vi "Init Galvo Commmand.vi"(8 "error in (no error)":errorcluster) -> (0 "error out":errorcluster)   [LabVIEW 2018]
uses:
  Controls/FGV Actions.ctl
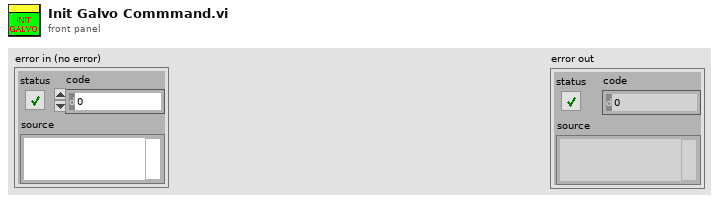
[diagram p1: front panel]
types:
  T1 = enum16{"Configure channels", "Write Scan Pattern", "Start Galvo Task", "Is Task Done?", "Stop Galvo", "Uninit", "Init: Calc scan pattern"}
  T2 = typedef "FGV Actions.ctl" = enum16{"Init", "Set", "Get", "Clear"}
  T3 = typedef "System Parameters.ctl" = cluster{"Optical Parameters":T4, "Vibratome":T5, "Table Stages":T6, "Imaging Parameter":T9, "Galvo HW Parameters":cluster{"Analog Out Channel":tag, "Min Voltage":dbl, "Max Voltage":dbl, "Pixel Clock Source":tag, "Sample Rate":dbl, "Line Clock Out Ch":tag}, "Alazar parameters":T11, "Mosaic Paramter":cluster{"X Axis":cluster{"Start [mm]":dbl, "Steps [pts]":u16, "End [mm]":dbl}, "Y Axis":cluster{"Start [mm]":dbl, "Steps [pts]":u16, "End [mm]":dbl}, "Scan Pattern":enum16{"Uni-directional", "Bi-Directional", "Spiral Out", "Spiral In"}, "Overlap Options":cluster{"Overlap Type":enum16{"No Overlap", "X Only", "Y Only", "X and Y"}, "Percent Overlap":u8, "Justify":enum16{"Start", "Center", "End"}}}, "Vibratome Axis":cluster{"Start [mm](next cut height)":dbl, "thick[um]":dbl, "#slices":dbl}}
  T4 = typedef "Optical Parameters.ctl" = cluster{"Obj. Focal Length [mm]":dbl, "Scan Lens EFL[mm]":dbl, "Tube Lens EFL[mm]":dbl, "Galvo V Range (+/-)":dbl, "Galvo Max Half Angle [Deg]":dbl, "Max Galvo Range[%]":dbl}
  T5 = typedef "Vibratome Parameters.ctl" = cluster{"Z Bottom [mm]":dbl, "Pre Cut Dwell [s]":dbl, "Blade Frequency [RPM]":u16, "Slice Speed [mm/s]":dbl, "Post Cut Dwell [s]":dbl, "Ramp Time [s]":dbl, "Start X [mm]":dbl, "Start Y [mm]":dbl, "Slice Length [mm]":dbl, "Slice Axis":enum16{"X Axis", "Y Axis", "Z Axis"}, "Controller VISA Ref":refnum<visa-resource-name>}
  T6 = typedef "Translation Stage Parameters.ctl" = cluster{"X Stage":T7, "Y Stage":T7, "Z Stage":T7}
  T7 = typedef "Translation Stage Cluster.ctl" = cluster{"Position":dbl, "Is.Enabled?":bool, "Is.Connected?":bool, "Device SN":string, "AccelerationMaximum":dbl, "VelocityMaximum":dbl, "Acceleration":dbl, "Velocity":dbl, "waitTimeout (ms)":i32, "Model":T8, "Is.Homed?":bool}
  T8 = typedef "Translation Stage Types.ctl" = enum16{"None", "Thorlabs LTS", "Thorlabs MLJ"}
  T9 = typedef "Imaging Parameters.ctl" = cluster{"Raster Scan Direction":T10, "Pixel Dwell Time [Clock Cycles]":u16, "Flyback Time [Clock Cycles]":u16, "XY Center [um]":cluster{"X":dbl, "Y":dbl}, "Pixel Step Size [um]":dbl, "XY Image Size":enum16{"32 x 32", "64 x 64", "128 x 128", "256 x 256", "512 x 512", "1024 x 1024", "2048 x 2048"}, "Custom":bool, "Custom Size":cluster{"X":u16, "Y":u16}, "Line Averages":u8}
  T10 = typedef "Scan Direction.ctl" = enum16{"Uni Directional", "Bi Directional", "None"}
  T11 = typedef "Alazar parameters.ctl" = cluster{"Trigger Settings":cluster{"General Trigger Settings":T12, "Trigger Engine 1":T13, "Trigger Engine 2":T13}, "Capture Clock":T14, "Device ID":T15, "Ch A Input Control":T16, "Ch B Input Control":T16, "Acq Settings":T17}
  T12 = typedef "General Trigger Settings.ctl" = cluster{"Trigger Operation":u32, "Coupling ID":u32, "Range ID":u32, "Delay":u32, "Timeout Ticks":u32, "Mode":u32, "Parameter":u32}
  T13 = typedef "Trigger Engine Controls.ctl" = cluster{"Trigger Engine":u32, "Source":u32, "Slope":u32, "Level":u32}
  T14 = typedef "Clock Controls.ctl" = cluster{"Sample Rate":u32, "Decimation":u32, "Source":u32, "Edge":u32}
  T15 = typedef "Alazar Device ID.ctl" = cluster{"System ID":u32, "Board ID":u32}
  T16 = typedef "Channel Input Controls.ctl" = cluster{"Channel":u8, "Coupling":u32, "Range":u32, "Impedance":u32}
  T17 = typedef "Alazar Acquisition Settings.ctl" = cluster{"Record Length":u32, "Offset":u32, "Records Per Buffer":u32, "Records Count (Records/Acq)":u32}
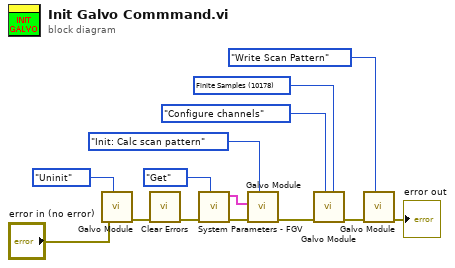
[diagram p0: block diagram]
diagram:
  w11 = 10178 items=["Finite Samples"=10178, "Continuous Samples"=10123, "Hardware Timed Single Point"=12522] ("sample mode")
  n1 = call "Galvo Module.vi"("Action"=T1."Uninit", "error in (no error)"="error in (no error)") -> ("error out"=w5:errorcluster)  [unwired: 8 in, 1 out]
  n2 = call <vilib>:"Clear Errors.vi"("error in (no error)"=w5) -> ("error out"=w3:errorcluster)  [unwired: 5 in, 1 out]
  n3 = call "System Parameters - FGV.vi"("Actions"=FGV_Actions."Get", "Error In"=w3) -> ("Error Out"=w6:errorcluster, "System Parameters"=w7:T3)  [unwired: 8 in]
  n4 = call "Galvo Module.vi"("Action"=T1."Init: Calc scan pattern", "error in (no error)"=w6, "System Parameters"=w7) -> ("error out"=w13:errorcluster)  [unwired: 7 in, 1 out]
  n5 = call "Galvo Module.vi"("sample mode"=w11, "Action"=T1."Configure channels", "error in (no error)"=w13) -> ("error out"=w14:errorcluster)  [unwired: 7 in, 1 out]
  n6 = call "Galvo Module.vi"("Action"=T1."Write Scan Pattern", "error in (no error)"=w14) -> ("error out"=→"error out":errorcluster)  [unwired: 8 in, 1 out]
